vi "sftp_append.vi"() -> ()   [LabVIEW 2013]
doc: "Illustrates how to append to a file using SFTP."
uses:
  libssh2/libssh2_init_default.vi
  libssh2/libssh2_session_handshake_tcp.vi
  libssh2/libssh2.lvlib
panel:
  out "file position before write":u64
  out "file position after write":u64
  out "filesize":u64
  out "file content":string
  in  "file":string="/"
  in  "append text":string="Lorem ipsum dolor sit amet, consetetur sadipscing elitr, sed diam nonumy eirmod tempor invidunt ut labore et dolore magna aliquyam erat, sed diam voluptua. At vero eos et accusam et justo duo dolores et ea rebum. Stet clita kasd gubergren, no sea takimata sanctus est Lorem ipsum dolor sit amet. Lorem ipsum dolor sit amet, consetetur sadipscing elitr, sed diam nonumy eirmod tempor invidunt ut labore et dolore magna aliquyam erat, sed diam voluptua. At vero eos et accusam et justo duo dolores et ea rebum. Stet clita kasd gubergren, no sea takimata sanctus est Lorem ipsum dolor sit amet. "
  out "error out":errorcluster
  in  "password":string
  in  "username":string
  in  "hostname":string
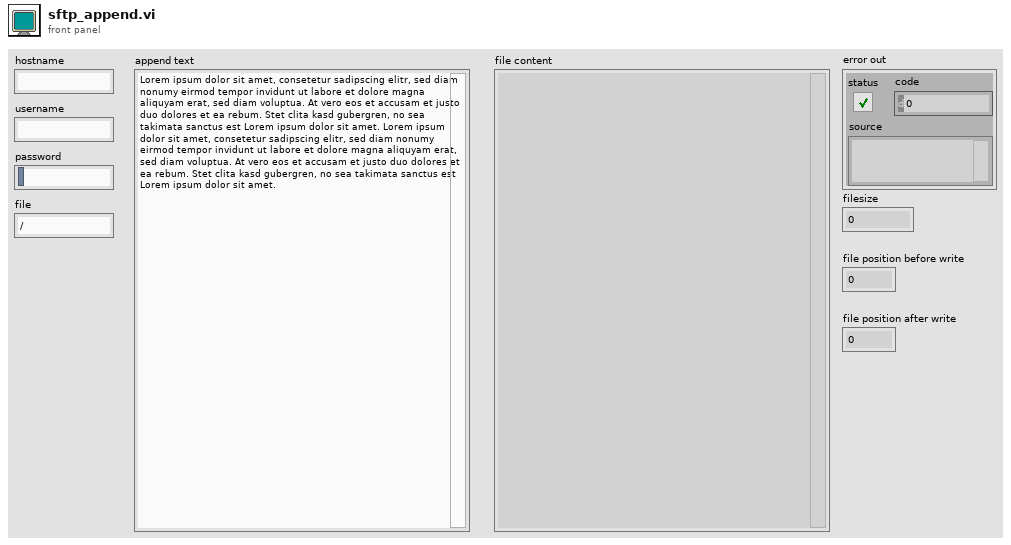
[diagram p1: front panel]
types:
  T1 = typedef "libssh2.lvlib/Session Refnum.ctl" = refnum<k1>
  T2 = typedef "libssh2.lvlib/SFTP Refnum.ctl" = refnum<k1>
  T3 = typedef "libssh2.lvlib/SFTP Handle Refnum.ctl" = refnum<k1>
  T4 = typedef "libssh2.lvlib/libssh2_sftp_attributes.ctl" = cluster{"flags":u32, "filesize":u64, "uid":u32, "gid":u32, "permissions":u32, "atime":u32, "mtime":u32}
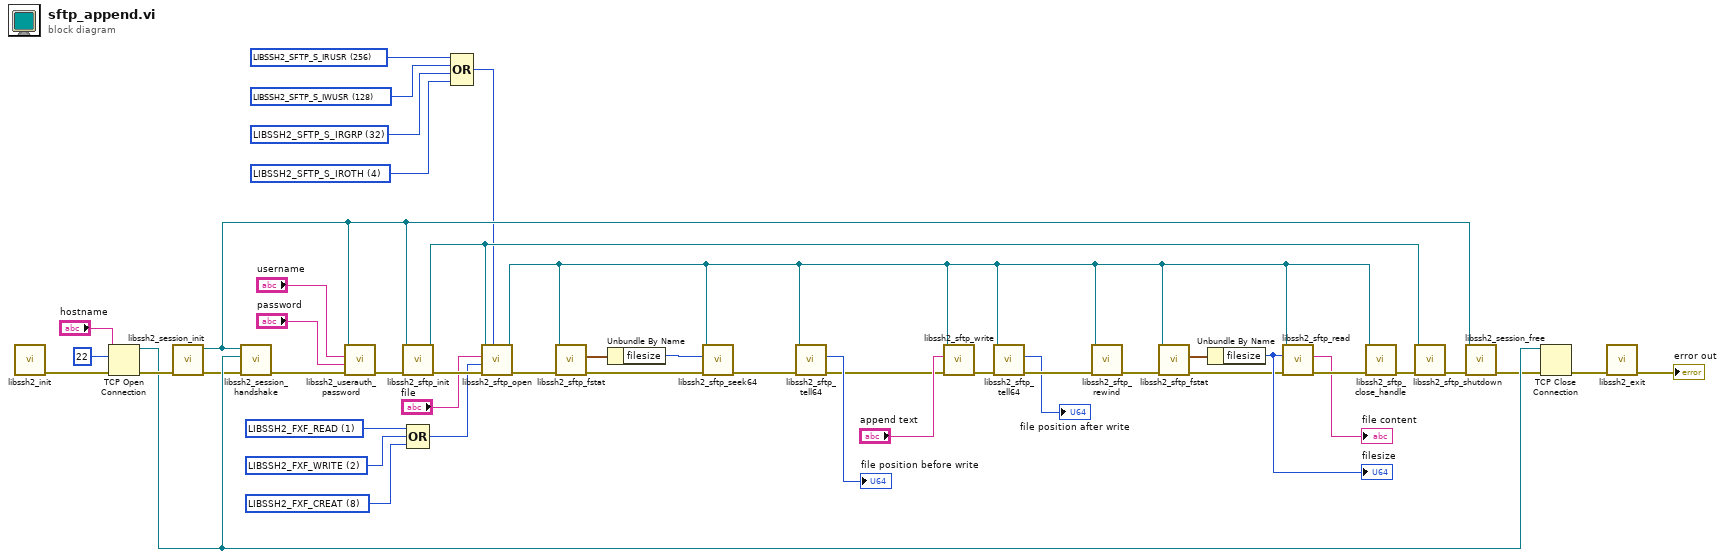
[diagram p0: block diagram]
diagram:
  w13 = u32 8 items=["LIBSSH2_FXF_READ"=1, "LIBSSH2_FXF_WRITE"=2, "LIBSSH2_FXF_APPEND"=4, "LIBSSH2_FXF_CREAT"=8, "LIBSSH2_FXF_TRUNC"=16, "LIBSSH2_FXF_EXCL"=32] ("flags")
  w21 = 4 items=["LIBSSH2_SFTP_S_IRWXU"=448, "LIBSSH2_SFTP_S_IRUSR"=256, "LIBSSH2_SFTP_S_IWUSR"=128, "LIBSSH2_SFTP_S_IXUSR"=64, "LIBSSH2_SFTP_S_IRWXG"=56, "LIBSSH2_SFTP_S_IRGRP"=32, "LIBSSH2_SFTP_S_IWGRP"=16, "LIBSSH2_SFTP_S_IXGRP"=8, "LIBSSH2_SFTP_S_IRWXO"=7, "LIBSSH2_SFTP_S_IROTH"=4, "LIBSSH2_SFTP_S_IWOTH"=2, "LIBSSH2_SFTP_S_IXOTH"=1] ("mode")
  w22 = 32 items=["LIBSSH2_SFTP_S_IRWXU"=448, "LIBSSH2_SFTP_S_IRUSR"=256, "LIBSSH2_SFTP_S_IWUSR"=128, "LIBSSH2_SFTP_S_IXUSR"=64, "LIBSSH2_SFTP_S_IRWXG"=56, "LIBSSH2_SFTP_S_IRGRP"=32, "LIBSSH2_SFTP_S_IWGRP"=16, "LIBSSH2_SFTP_S_IXGRP"=8, "LIBSSH2_SFTP_S_IRWXO"=7, "LIBSSH2_SFTP_S_IROTH"=4, "LIBSSH2_SFTP_S_IWOTH"=2, "LIBSSH2_SFTP_S_IXOTH"=1] ("mode")
  w23 = 128 items=["LIBSSH2_SFTP_S_IRWXU"=448, "LIBSSH2_SFTP_S_IRUSR"=256, "LIBSSH2_SFTP_S_IWUSR"=128, "LIBSSH2_SFTP_S_IXUSR"=64, "LIBSSH2_SFTP_S_IRWXG"=56, "LIBSSH2_SFTP_S_IRGRP"=32, "LIBSSH2_SFTP_S_IWGRP"=16, "LIBSSH2_SFTP_S_IXGRP"=8, "LIBSSH2_SFTP_S_IRWXO"=7, "LIBSSH2_SFTP_S_IROTH"=4, "LIBSSH2_SFTP_S_IWOTH"=2, "LIBSSH2_SFTP_S_IXOTH"=1] ("mode")
  w24 = 256 items=["LIBSSH2_SFTP_S_IRWXU"=448, "LIBSSH2_SFTP_S_IRUSR"=256, "LIBSSH2_SFTP_S_IWUSR"=128, "LIBSSH2_SFTP_S_IXUSR"=64, "LIBSSH2_SFTP_S_IRWXG"=56, "LIBSSH2_SFTP_S_IRGRP"=32, "LIBSSH2_SFTP_S_IWGRP"=16, "LIBSSH2_SFTP_S_IXGRP"=8, "LIBSSH2_SFTP_S_IRWXO"=7, "LIBSSH2_SFTP_S_IROTH"=4, "LIBSSH2_SFTP_S_IWOTH"=2, "LIBSSH2_SFTP_S_IXOTH"=1] ("mode")
  w26 = u32 2 items=["LIBSSH2_FXF_READ"=1, "LIBSSH2_FXF_WRITE"=2, "LIBSSH2_FXF_APPEND"=4, "LIBSSH2_FXF_CREAT"=8, "LIBSSH2_FXF_TRUNC"=16, "LIBSSH2_FXF_EXCL"=32] ("flags")
  w27 = u32 1 items=["LIBSSH2_FXF_READ"=1, "LIBSSH2_FXF_WRITE"=2, "LIBSSH2_FXF_APPEND"=4, "LIBSSH2_FXF_CREAT"=8, "LIBSSH2_FXF_TRUNC"=16, "LIBSSH2_FXF_EXCL"=32] ("flags")
  n1 = call-poly "libssh2_init.vi"() -> ("error out"=w45:errorcluster)  [unwired: 11 in]
  n2 = TCP Open Connection(address="hostname", remote port or service name=u16 22, error in (no error)=w45) -> (connection ID=w43:refnum<k5>, error out=w44:errorcluster)  [unwired: 2 in]
  n3 = call "libssh2_session_init.vi"("error in (no error)"=w44) -> ("error out"=w42:errorcluster, "session"=w35:T1)  [unwired: 9 in]
  n4 = call-poly "libssh2_session_handshake.vi"("error in (no error)"=w42, "tcp connection"=w43, "session"=w35) -> ("error out"=w46:errorcluster)  [unwired: 8 in]
  n5 = call "libssh2_userauth_password.vi"("error in (no error)"=w46, "password"="password", "username"="username", "session"=w35) -> ("error out"=w39:errorcluster)  [unwired: 7 in]
  n6 = call "libssh2_sftp_init.vi"("error in (no error)"=w39, "session"=w35) -> ("error out"=w31:errorcluster, "sftp"=w30:T2)  [unwired: 8 in]
  n7 = Compound Arithmetic op=OR(w27, w26, w13) -> (w25:u32)
  n8 = Compound Arithmetic op=OR(w24, w23, w22, w21) -> (w20:i32)
  n9 = call "libssh2_sftp_open.vi"("mode"=w20, "error in (no error)"=w31, "flags"=w25, "path"="file", "sftp"=w30) -> ("error out"=w19:errorcluster, "sftp handle"=w1:T3)  [unwired: 5 in]
  n10 = call "libssh2_sftp_fstat.vi"("error in (no error)"=w19, "sftp handle"=w1) -> ("error out"=w18:errorcluster, "attributes out"=w17:T4)  [unwired: 8 in]
  n11 = Unbundle By Name(w17) -> ("filesize"=w16:u64)
  n12 = call "libssh2_sftp_seek64.vi"("error in (no error)"=w18, "offset"=w16, "sftp handle"=w1) -> ("error out"=w3:errorcluster)  [unwired: 8 in]
  n13 = call "libssh2_sftp_tell64.vi"("error in (no error)"=w3, "sftp handle"=w1) -> ("error out"=w2:errorcluster, "offset"=→"file position before write":u64)  [unwired: 8 in]
  n14 = call "libssh2_sftp_write.vi"("error in (no error)"=w2, "buffer"="append text", "sftp handle"=w1) -> ("error out"=w15:errorcluster)  [unwired: 7 in, 1 out]
  n15 = call "libssh2_sftp_tell64.vi"("error in (no error)"=w15, "sftp handle"=w1) -> ("error out"=w6:errorcluster, "offset"=→"file position after write":u64)  [unwired: 8 in]
  n16 = call "libssh2_sftp_rewind.vi"("error in (no error)"=w6, "sftp handle"=w1) -> ("error out"=w9:errorcluster)  [unwired: 9 in]
  n17 = call "libssh2_sftp_fstat.vi"("error in (no error)"=w9, "sftp handle"=w1) -> ("error out"=w8:errorcluster, "attributes out"=w11:T4)  [unwired: 8 in]
  n18 = Unbundle By Name(w11) -> ("filesize"=w10:u64)
  "filesize" <- w10
  n19 = call "libssh2_sftp_read.vi"("error in (no error)"=w8, "buffer maxlen"=w10, "sftp handle"=w1) -> ("error out"=w12:errorcluster, "buffer"=→"file content":string)  [unwired: 6 in, 1 out]
  n20 = call "libssh2_sftp_close_handle.vi"("error in (no error)"=w12, "sftp handle"=w1) -> ("error out"=w28:errorcluster)  [unwired: 9 in]
  n21 = call "libssh2_sftp_shutdown.vi"("error in (no error)"=w28, "sftp"=w30) -> ("error out"=w32:errorcluster)  [unwired: 9 in]
  n22 = call "libssh2_session_free.vi"("error in (no error)"=w32, "session"=w35) -> ("error out"=w34:errorcluster)  [unwired: 9 in]
  n23 = TCP Close Connection(connection ID=w43, error in (no error)=w34) -> (error out=w33:errorcluster)  [unwired: 1 in, 1 out]
  n24 = call "libssh2_exit.vi"("error in (no error)"=w33) -> ("error out"=→"error out":errorcluster)  [unwired: 10 in]
